vi "Make Observer.vi"(1 "To be an Observer":refnum<class "Send.lvclass">) -> (0 "Observer":refnum<class "Observer.lvclass">)   [LabVIEW 2011, in "Messenging.lvlib" / "Observer.lvclass"]
uses:
  Observer.lvclass
  Send/Send.lvclass
  SendMultiple/ObserverSet.lvclass
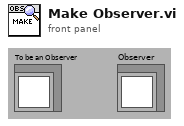
[diagram p1: front panel]
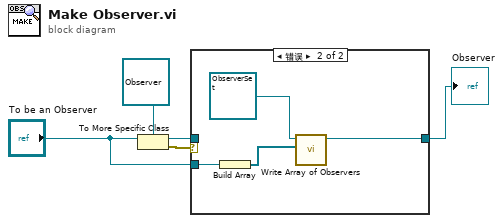
[diagram p0: block diagram]
diagram:
  n1 = To More Specific Class(target class=refnum<class "Observer.lvclass"> refnum ("Observer"), reference="To be an Observer") -> (specific class reference=w4:refnum<class "Observer.lvclass">, error out=w3:errorcluster)  [unwired: 1 in]
  n2 = case shown="错误" w3 {
    tunnel: w4 -> [w6 _]
    tunnel: [w6 w7] -> w5
    tunnel: "To be an Observer" -> [_ w10]
    frame No Error {
    }
    frame Error {
      n3 = Build Array(w10) -> (w9:refnum<class "Send.lvclass">[])
      n4 = call "Write Array of Observers.vi"("Array of Observers"=w9, "ObserverSet.lvclass in"=refnum<class "ObserverSet.lvclass"> refnum ("Messenging.lvlib:ObserverSet.lvclass")) -> ("ObserverSet.lvclass out"=w7:refnum<class "ObserverSet.lvclass">)  [unwired: 1 in, 8 out]
    }
  }
  "Observer" <- w5
